vi "Torque, Load, and Efficiency (Air Gap, 1 Motor with IC).vi"(0 "phase voltage waveforms":waveform(dbl)[](array[waveform]), 1 "fundamental frequency [Hz]":dbl=50.0, 2 "reset? (F)":bool, 5 "current waveforms":waveform(dbl)[](array[waveform]), 7 "speed [RPM]":dbl, 9 "initial conditions":T1, 11 "error in (no error)":errorcluster, 12 "nameplate information":T2, 13 "total input active power [W]":dbl, 14 "stator resistance [ohms]":dbl) -> (3 "torque waveform [Nm]":waveform(dbl), 4 "torque [Nm]":dbl, 6 "load [kW]":dbl, 8 "efficiency [%]":dbl, 10 "final conditions":T1, 15 "error out":errorcluster)   [LabVIEW 2014, in "NI_EP_Motor Monitoring.lvlib"]
doc: "Calculates the torque, load, and efficiency values based on the motor nameplate information. You must manually select the polymorphic instance you want to use."
uses:
  <vilib>/addons/Electrical Power/Motor Monitoring/NI_EP_Motor Monitoring.lvlib
  <vilib>/addons/Electrical Power/Motor Monitoring/subVIs/ep_Initial Conditions for Air Gap.ctl
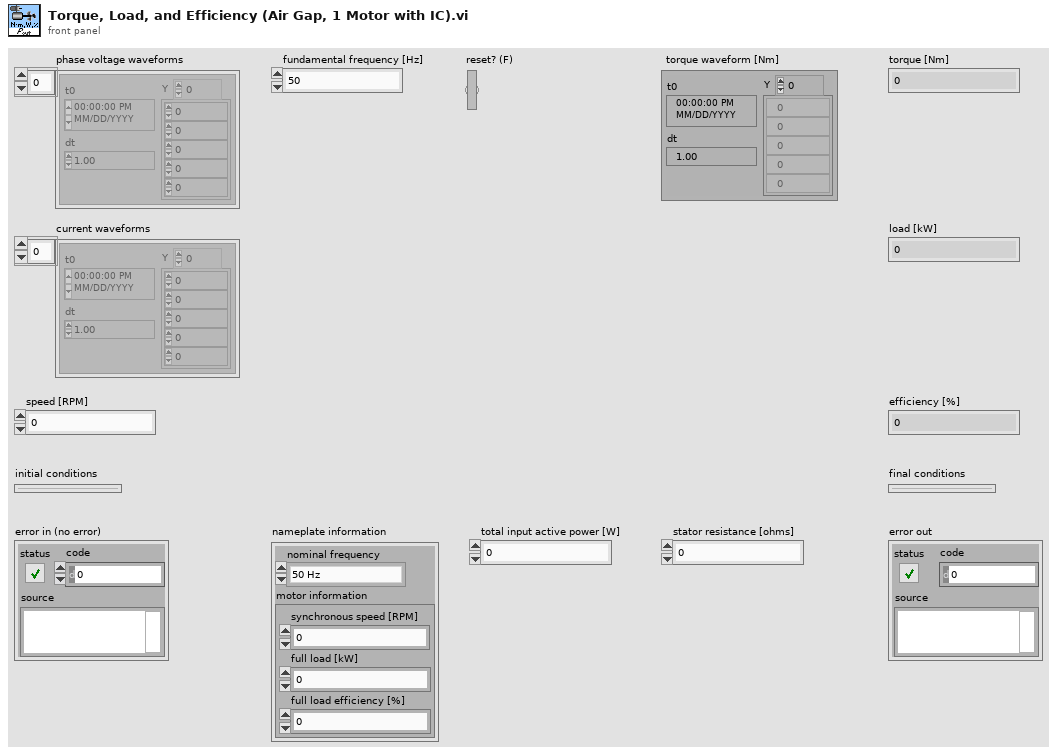
[diagram p1: front panel]
types:
  T1 = typedef "NI_EP_Motor Monitoring.lvlib/ep_Initial Conditions for Air Gap.ctl" = cluster{"integration state in A":cluster{"initial value":dbl, "initial integration":dbl}, "integration state in B":cluster{"initial value":dbl, "initial integration":dbl}, "integrated state A":dbl[], "integrated state B":dbl[], "previous length":i32, "loss and polepair":cluster{"Pstray [W]":dbl, "Pfric [W]":dbl, "Polepair #":i32, "synchronous speed [RPM]":dbl}, "expected timestamp":timestamp}
  T2 = cluster{"nominal frequency":enum16{"50 Hz", "60 Hz"}, "motor information":cluster{"synchronous speed [RPM]":dbl, "full load [kW]":dbl, "full load efficiency [%]":dbl}}
  T3 = cluster{"synchronous speed [RPM]":dbl, "full load [kW]":dbl, "full load efficiency [%]":dbl}
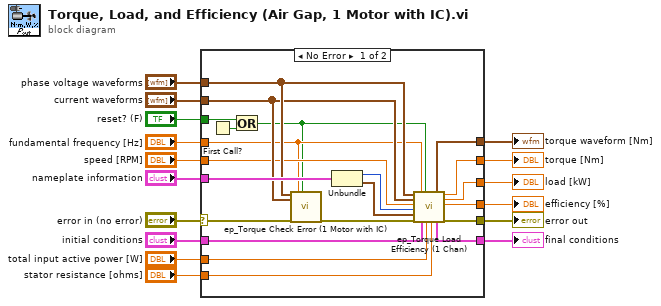
[diagram p0: block diagram]
diagram:
  n1 = case shown="No Error" "error in (no error)" {
    selector: "error in (no error)" -> [w22 w38]
    tunnel: [w32 w38] -> w15
    tunnel: "reset? (F)" -> [w36 _]
    tunnel: "fundamental frequency [Hz]" -> [w18 _]
    tunnel: "nameplate information" -> [w35 _]
    tunnel: "current waveforms" -> [w20 _]
    tunnel: "phase voltage waveforms" -> [w21 _]
    tunnel: [w31 _] -> w1
    tunnel: [w30 _] -> w4
    tunnel: [w29 _] -> w2
    tunnel: [w28 _] -> w3
    tunnel: "speed [RPM]" -> [w19 _]
    tunnel: "stator resistance [ohms]" -> [w27 _]
    tunnel: "total input active power [W]" -> [w26 _]
    tunnel: "initial conditions" -> [w25 _]
    tunnel: [w24 _] -> w5
    frame No Error {
      n2 = First Call?() -> (First Call?: T/F=w37:bool)
      n3 = Or(x=w36, y=w37) -> (x .or. y?=w17:bool)
      n4 = call <vilib>:"ep_Torque Check Error (1 Motor with IC).vi"("phase voltage waveforms"=w21, "current waveforms"=w20, "error in (no error)"=w22, "fundamental frequency [Hz]"=w18, "reset? (F)"=w17) -> ("error out"=w23:errorcluster)  [unwired: 14 in]
      n5 = Unbundle(w35) -> ("nominal frequency"=w34:enum16{"50 Hz", "60 Hz"}, "motor information"=w33:T3)
      n6 = call <vilib>:"ep_Torque Load Efficiency (1 Chan).vi"("phase voltage waveforms"=w21, "current waveforms"=w20, "speed [RPM]"=w19, "nominal frequency"=w34, "motor information"=w33, "error in (no error)"=w23, "fundamental frequency [Hz]"=w18, "initial conditions"=w25, "reset? (F)"=w17, "total input active power [W]"=w26, "stator resistance [ohms]"=w27) -> ("torque waveform [Nm]"=w31:waveform(dbl), "final conditions"=w24:T1, "torque [Nm]"=w30:dbl, "load [kW]"=w29:dbl, "efficiency [%]"=w28:dbl, "error out"=w32:errorcluster)  [unwired: 3 in]
    }
    frame Error {
    }
  }
  "error out" <- w15
  "torque waveform [Nm]" <- w1
  "torque [Nm]" <- w4
  "load [kW]" <- w2
  "efficiency [%]" <- w3
  "final conditions" <- w5
